vi "GetDataSource.vi"(10 "data source id":string, 11 "data sources in":T1[](array[typedef])) -> (1 "found":bool, 2 "DataSource":T1, 3 "data sources out":T1[](array[typedef]))   [LabVIEW 2017, in "DeviceModelHelpers.lvlib"]
uses:
  <vilib>/addons/InsightCM/Utilities/DeviceModelHelpers/DeviceModelHelpers.lvlib
  <vilib>/addons/InsightCM/MessageBus/Base/controls/DataSource.ctl
  <vilib>/addons/InsightCM/MessageBus/Base/controls/KeyValuePair.ctl
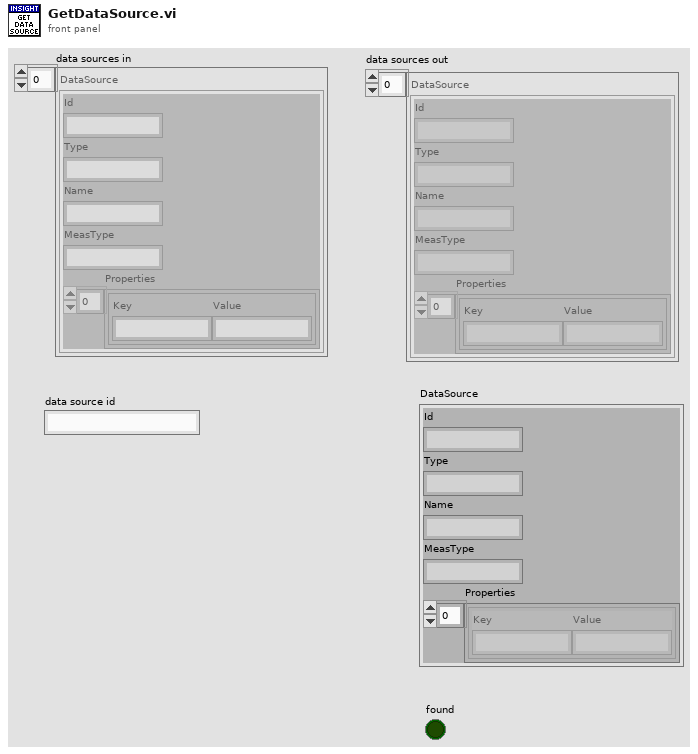
[diagram p1: front panel]
types:
  T1 = typedef "DataSource.ctl" = cluster{"Id":string, "Type":string, "Name":string, "MeasType":string, "Properties":T2[]}
  T2 = typedef "KeyValuePair.ctl" = cluster{"Key":string, "Value":string}
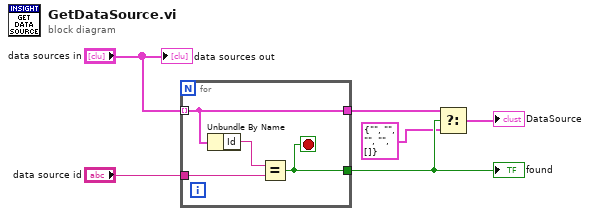
[diagram p0: block diagram]
diagram:
  n1 = for {
    tunnel: "data sources in" -> [w8] mode=indexing
    tunnel: "data source id" -> [w9]
    tunnel: [w8] -> w4
    tunnel: [w7] -> w5
    stop <- w7 stop-if-true
    n2 = Unbundle By Name(w8) -> ("Id"=w10:string)
    n3 = Equal?(x=w10, y=w9) -> (x = y?=w7:bool)
  }
  "found" <- w5
  n4 = Select(t=w4, s=w5, f=T1 {"Id"="", "Type"="", "Name"="", "MeasType"="", "Properties"=[]} ("DataSource")) -> (s? t:f=→"DataSource":T1)
  "data sources out" <- "data sources in"
